vi "LL_GET Object (Core).vi"(7 "output file":path=path "", 8 "error in (no error)":errorcluster, 9 "Bucket":string, 10 "Path and query string":string="/", 11 "Headers":T2[](array[typedef])) -> (0 "error out":errorcluster, 1 "Call Result":T1, 2 "Response body":string, 3 "Response header":string)   [LabVIEW 2011, in "LV Interface for Amazon S3.lvlib"]
doc: "This core implementation of the GET operation may be used to implement special requests or API calls not present in this toolkit. You can set the output file input to a valid path to save the response body to a file."
uses:
  LV Interface for Amazon S3.lvlib
  Typedefs/AMZ_S3_HTTP Header-Value pair.ctl
  Typedefs/AMZ_S3_Call Results.ctl
  <vilib>/httpClient/LabVIEWHTTPClient.lvlib
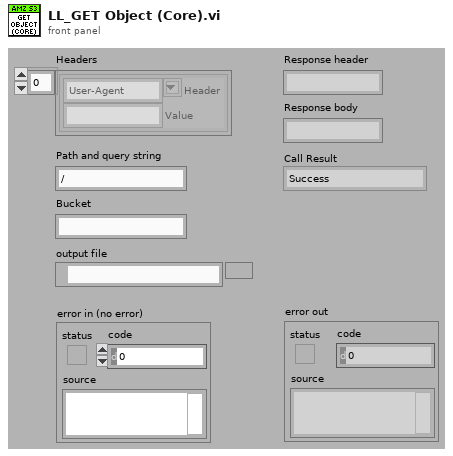
[diagram p1: front panel]
types:
  T1 = typedef "LV Interface for Amazon S3.lvlib/AMZ_S3_Call Results.ctl" = enum16{"Success", "UndefinedError", "AccessDenied", "AccountProblem", "AmbiguousGrantByEmailAddress", "BadDigest", "BucketAlreadyExists", "BucketAlreadyOwnedByYou", "BucketNotEmpty", "CredentialsNotSupported", "CrossLocationLoggingProhibited", "EntityTooSmall", "EntityTooLarge", "ExpiredToken", "IllegalVersioningConfigurationException", "IncompleteBody", "IncorrectNumberOfFilesInPostRequest", "InlineDataTooLarge", "InternalError", "InvalidAccessKeyId", "InvalidAddressingHeader", "InvalidArgument", "InvalidBucketName", "InvalidDigest", "InvalidLocationConstraint", "InvalidPart", "InvalidPartOrder", "InvalidPayer", "InvalidPolicyDocument", "InvalidRange", "InvalidSecurity", "InvalidSOAPRequest", "InvalidStorageClass", "InvalidTargetBucketForLogging", "InvalidToken", "InvalidURI", "KeyTooLong", "MalformedACLError", "MalformedPOSTRequest", "MalformedXML", "MaxMessageLengthExceeded", "MaxPostPreDataLengthExceededError", "MetadataTooLarge", "MethodNotAllowed", "MissingAttachment", "MissingContentLength", "MissingRequestBodyError", "MissingSecurityElement", "MissingSecurityHeader", "NoLoggingStatusForKey", "NoSuchBucket", "NoSuchKey", "NoSuchUpload", "NoSuchVersion", "NotImplemented", "NotSignedUp", "OperationAborted", "PermanentRedirect", "PreconditionFailed", "Redirect", "RequestIsNotMultiPartContent", "RequestTimeout", "RequestTimeTooSkewed", "RequestTorrentOfBucketError", "SignatureDoesNotMatch", "SlowDown", "TemporaryRedirect", "TokenRefreshRequired", "TooManyBuckets", "UnexpectedContent", "UnresolvableGrantByEmailAddress", "UserKeyMustBeSpecified", "LabVIEWError"}
  T2 = typedef "LV Interface for Amazon S3.lvlib/AMZ_S3_HTTP Header-Value pair.ctl" = cluster{"Header":string, "Value":string}
  T3 = typedef "LabVIEWHTTPClient.lvlib/ClientHandle.ctl" = refnum<k1>
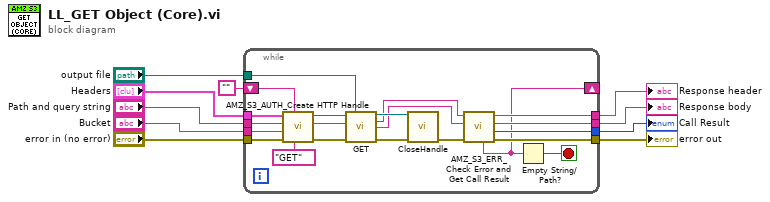
[diagram p0: block diagram]
diagram:
  n1 = while {
    tunnel: "Bucket" -> [w31]
    tunnel: "Path and query string" -> [w30]
    tunnel: "Headers" -> [w29]
    tunnel: "error in (no error)" -> [w28]
    tunnel: [w18] -> w6
    tunnel: [w17] -> w5
    tunnel: [w16] -> w4
    tunnel: [w15] -> w3
    shift-right: [w12] -> _
    shift-left: "" -> [w13]
    tunnel: "output file" -> [w11]
    stop <- w14 stop-if-true
    n2 = call "AMZ_S3_AUTH_Create HTTP Handle.vi"("HTTP-Verb"="GET", "Redirect endpoint"=w13, "error in (no error)"=w28, "Bucket"=w31, "Path and query string"=w30, "Headers"=w29) -> ("error out"=w26:errorcluster, "URL"=w24:string, "client handle out"=w25:T3)  [unwired: 3 in]
    n3 = call <vilib>:"GET.vi"("client handle"=w25, "output file"=w11, "url"=w24, "error in (no error)"=w26) -> ("client handle out"=w22:T3, "headers"=w20:string, "body"=w19:string, "error out"=w23:errorcluster)  [unwired: 8 in]
    n4 = call <vilib>:"CloseHandle.vi"("client handle"=w22, "error in (no error)"=w23) -> ("error out"=w21:errorcluster)  [unwired: 13 in]
    n5 = call "AMZ_S3_ERR_Check Error and Get Call Result.vi"("error in (no error)"=w21, "Response body"=w19, "Response header"=w20) -> ("error out"=w15:errorcluster, "Call Result"=w16:T1, "Response body dup"=w17:string, "Response header dup"=w18:string, "Redirect endpoint"=w12:string)  [unwired: 4 in]
    n6 = Empty String/Path?(string/path=w12) -> (empty?=w14:bool)
  }
  "Response header" <- w6
  "Response body" <- w5
  "Call Result" <- w4
  "error out" <- w3
